vi "Store Configuration Parameters.vi"(8 "error in (no error)":errorcluster, 10 "refnum":T1, 11 "Example Configuration Dialog in":refnum<class "Controller Configuration.lvclass">) -> (0 "error out":errorcluster, 2 "refnum out":T1, 3 "Example Configuration Dialog out":refnum<class "Controller Configuration.lvclass">)   [LabVIEW 2026, in "Msmt Configuration.lvlib" / "Controller Configuration.lvclass"]
uses:
  Controller Configuration.lvclass
  <vilib>/Utility/config.llb/Config Data RefNum.ctl
  Controller Configuration.lvclass/Controller Configuration.ctl
  configuration/Configuration.lvclass
  <vilib>/Utility/config.llb/NI_LVConfig.lvlib
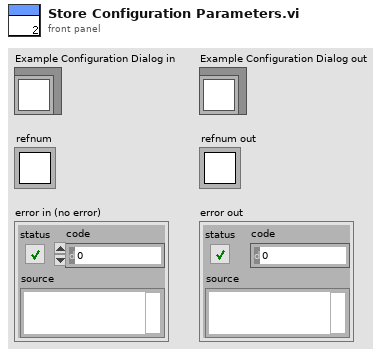
[diagram p1: front panel]
types:
  T1 = typedef "NI_LVConfig.lvlib/Config Data RefNum.ctl" = refnum<k1>
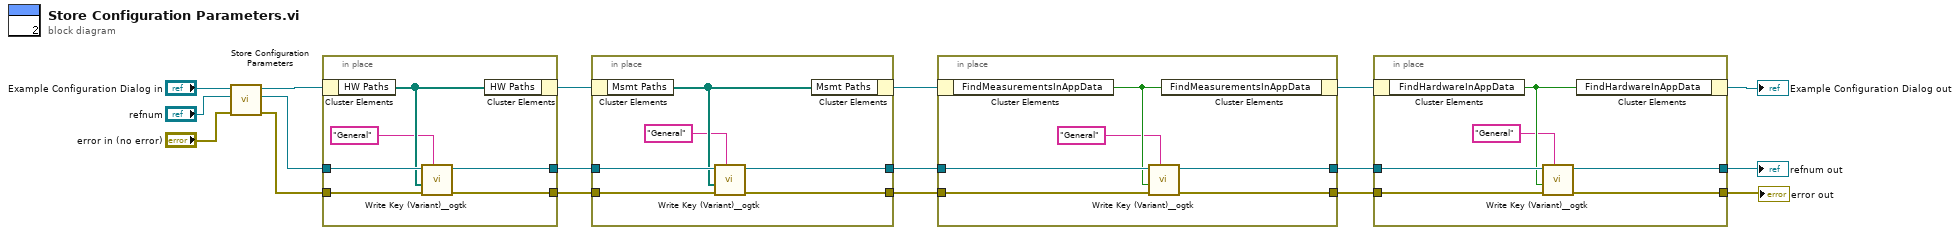
[diagram p0: block diagram]
diagram:
  n1 = call-parent "Store Configuration Parameters.vi"("error in (no error)"="error in (no error)", "refnum"="refnum", "Configuration in"="Example Configuration Dialog in") -> ("error out"=w14:errorcluster, "refnum out"=w15:T1, "Configuration out"=w13:refnum<class "Controller Configuration.lvclass">)  [unwired: 6 in]
  n2 = in-place "In Place Element Structure" {
    in-place-border: w15 -> [w24]
    in-place-border: w14 -> [w23]
    in-place-border: [w20] -> w11
    in-place-border: [w21] -> w12
    n3 = in-place-cluster #1(w13) -> ("HW Paths"=w22:path[])
    n4 = call <userlib>:"Write Key (Variant)__ogtk.vi"("section"="General", "error in (no error)"=w23, "key-value"=w22, "refnum"=w24) -> ("error out"=w20:errorcluster, "refnum out"=w21:T1)  [unwired: 6 in]
    n5 = in-place-cluster #1("HW Paths"=w22) -> (w10:refnum<class "Controller Configuration.lvclass">)
  }
  n6 = in-place "In Place Element Structure" {
    in-place-border: w12 -> [w30]
    in-place-border: w11 -> [w29]
    in-place-border: [w26] -> w4
    in-place-border: [w25] -> w5
    n7 = in-place-cluster #2(w10) -> ("Msmt Paths"=w28:path[])
    n8 = call <userlib>:"Write Key (Variant)__ogtk.vi"("section"="General", "error in (no error)"=w29, "key-value"=w28, "refnum"=w30) -> ("error out"=w26:errorcluster, "refnum out"=w25:T1)  [unwired: 6 in]
    n9 = in-place-cluster #2("Msmt Paths"=w28) -> (w6:refnum<class "Controller Configuration.lvclass">)
  }
  n10 = in-place "In Place Element Structure" {
    in-place-border: w5 -> [w36]
    in-place-border: w4 -> [w35]
    in-place-border: [w32] -> w8
    in-place-border: [w33] -> w7
    n11 = in-place-cluster #3(w6) -> ("FindMeasurementsInAppData"=w34:bool)
    n12 = call <userlib>:"Write Key (Variant)__ogtk.vi"("section"="General", "error in (no error)"=w35, "key-value"=w34, "refnum"=w36) -> ("error out"=w32:errorcluster, "refnum out"=w33:T1)  [unwired: 6 in]
    n13 = in-place-cluster #3("FindMeasurementsInAppData"=w34) -> (w9:refnum<class "Controller Configuration.lvclass">)
  }
  n14 = in-place "In Place Element Structure" {
    in-place-border: w7 -> [w42]
    in-place-border: w8 -> [w41]
    in-place-border: [w38] -> w1
    in-place-border: [w37] -> w2
    n15 = in-place-cluster #4(w9) -> ("FindHardwareInAppData"=w40:bool)
    n16 = call <userlib>:"Write Key (Variant)__ogtk.vi"("section"="General", "error in (no error)"=w41, "key-value"=w40, "refnum"=w42) -> ("error out"=w38:errorcluster, "refnum out"=w37:T1)  [unwired: 6 in]
    n17 = in-place-cluster #4("FindHardwareInAppData"=w40) -> (→"Example Configuration Dialog out":refnum<class "Controller Configuration.lvclass">)
  }
  "error out" <- w1
  "refnum out" <- w2
